vi "Finite Sample Start.vi"(0 "Arduino Resource":T1={"VISA resource"="", "Board Type"=enum."Arduino Uno", "Connection Type"=enum."USB / Serial", "Bytes Per Packet (15)"=15}, 5 "Analog Input Pin":u8, 7 "Acquition Speed (HZ)":u16, 9 "Number of Samples":u16, 11 "error in":errorcluster) -> (4 "Arduino Resource":T1={"VISA resource"="", "Board Type"=enum."Arduino Uno", "Connection Type"=enum."USB / Serial", "Bytes Per Packet (15)"=15}, 15 "error out":errorcluster)   [LabVIEW 2011, in "LabVIEW Interface for Arduino.lvlib"]
doc: "This VI configures and starts a finite execution on the Arduino. After this VI is run the arduino will start to output data to the serial port continuously until the number of samples set is reached."
uses:
  LabVIEW Interface for Arduino.lvlib
  Private/Type Defs/Arduino Resource.ctl
  Private/Type Defs/Board Type.ctl
  Private/Type Defs/Command.ctl
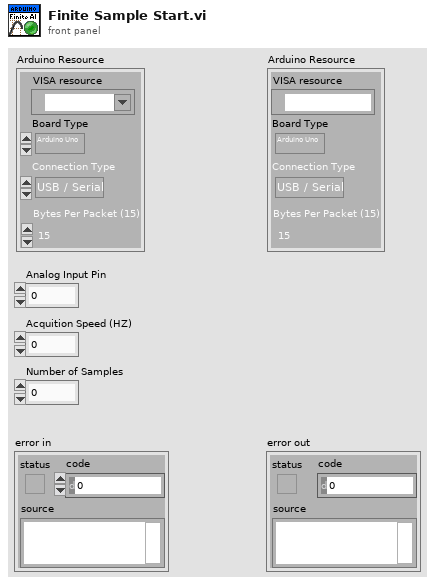
[diagram p1: front panel]
types:
  T1 = typedef "LabVIEW Interface for Arduino.lvlib/Arduino Resource.ctl" = cluster{"VISA resource":refnum<visa-resource-name>, "Board Type":T2, "Connection Type":enum8{"USB / Serial"}, "Bytes Per Packet (15)":u8}
  T2 = typedef "LabVIEW Interface for Arduino.lvlib/Board Type.ctl" = enum16{"Arduino Uno", "Dimuelanove w/Atmega 328", "Mega 2560", "Chipkit Uno32", "Chipkit Max32"}
  T3 = typedef "LabVIEW Interface for Arduino.lvlib/Command.ctl" = enum8{"setArduinoMode", "flushSerial", "setPinMode", "digitalWritePin", "digitalWritePort", "tone", "digitalReadPin", "digitalReadPort", "analogReadPin", "analogReadPort", "pwmWritePin", "pwmWritePort", "sevenSegment_Configure", "sevenSegment_Write", "I2C Init", "I2C Write", "I2C Read", "SPI Init", "SPI Set Bit Order", "SPI Set Clock Divider", "SPI Set Data Mode", "SPI Send / Receive", "SPI Close", "Servo Set Num Servos", "Servo Config Servo", "Servo Write Angle", "Servo Read Angle", "Servo Write Pulse Width", "Servo Read Pulse Width", "Servo Detach", "LCD Init", "LCD Set Size", "LCD Set Cursor Mode", "LCD Clear", "LCD Set Cursor Position", "LCD Print", "LCD Display Power", "LCD Scroll Display", "LCD Autoscroll", "LCD Print Direction", "LCD Create Custom Char", "LCD Print Custom Char", "contAcqOn", "contAcqOff", "getFirmwareVersion", "FiniteSampleStart"}
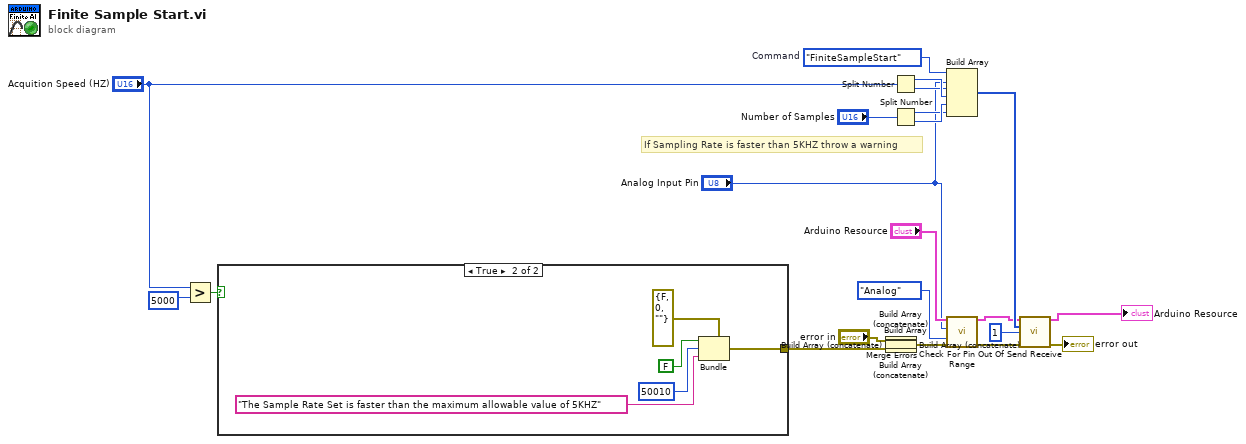
[diagram p0: block diagram]
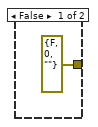
[diagram p2: hidden frame]
diagram:
  w25 = Command."FiniteSampleStart"  # Command
  # "If Sampling Rate is faster than 5KHZ throw a warning"
  n1 = Greater?(x="Acquition Speed (HZ)", y=u16 5000) -> (0:w11:bool)
  n2 = case shown="True" w11 {
    tunnel: [errorcluster {"status"=FALSE, "code"=0, "source"=""} ("error out") w28] -> w6
    frame False {
    }
    frame True {
      n3 = Bundle(cluster=errorcluster {"status"=FALSE, "code"=0, "source"=""} ("error out"), "status"=FALSE, "code"=50010, "source"="The Sample Rate Set is faster than the maximum allowable value of 5KHZ") -> (w28:errorcluster)
    }
  }
  n4 = Build Array("error in", w6) -> (w5:errorcluster[])
  n5 = Build Array (concatenate)(w5) -> (w4:errorcluster[])
  n6 = Build Array (concatenate)(w4) -> (w3:errorcluster[])
  n7 = Build Array (concatenate)(w3) -> (w2:errorcluster[])
  n8 = Build Array (concatenate)(w2) -> (w1:errorcluster[])
  n9 = Merge Errors(w1) -> (w8:errorcluster)
  n10 = Split Number(x="Acquition Speed (HZ)") -> (hi(x)=w24:u8, lo(x)=w23:u8)
  n11 = Split Number(x="Number of Samples") -> (hi(x)=w20:u8, lo(x)=w21:u8)
  n12 = Build Array(w25, "Analog Input Pin", w23, w24, w21, w20) -> (w19:u8[])
  n13 = call "Check For Pin Out Of Range.vi"("Arduino Resource"="Arduino Resource", "User Pin Number"="Analog Input Pin", "Pin Type"=enum16{"Analog", "Digital"}."Analog", "error in"=w8) -> ("Arduino Resource"=w16:T1, "error out"=w18:errorcluster)  [unwired: 10 in]
  n14 = call "Send Receive.vi"("Arduino Resource"=w16, "Data"=w19, "Bytes To Read (0)"=u8 1, "error in"=w18) -> ("Arduino Resource"=→"Arduino Resource":T1, "error out"=→"error out":errorcluster)  [unwired: 9 in, 1 out]
